vi "rerunSummary.vi"() -> ()   [LabVIEW 2012]
uses:
  <vilib>/addons/database/Auxilliary.llb/DB Tools Cursor Type.ctl
  <vilib>/addons/database/Connection.llb/DB Tools Open Connec (Path).vi
  <vilib>/addons/database/Connection.llb/Conn Execute.vi
  <vilib>/addons/database/Recordset.llb/Rec Destroy - Connection.vi
  <vilib>/addons/database/NI_Database_API.lvlib
panel:
  in  "machine":string
  out "error out":errorcluster
  in  "path":path
  in  "input cluster 2":T1
  out "output cluster":T1
  out "concatenated string":string
  out "concatenated string 2":string
  out "filenames":string[](array[string])
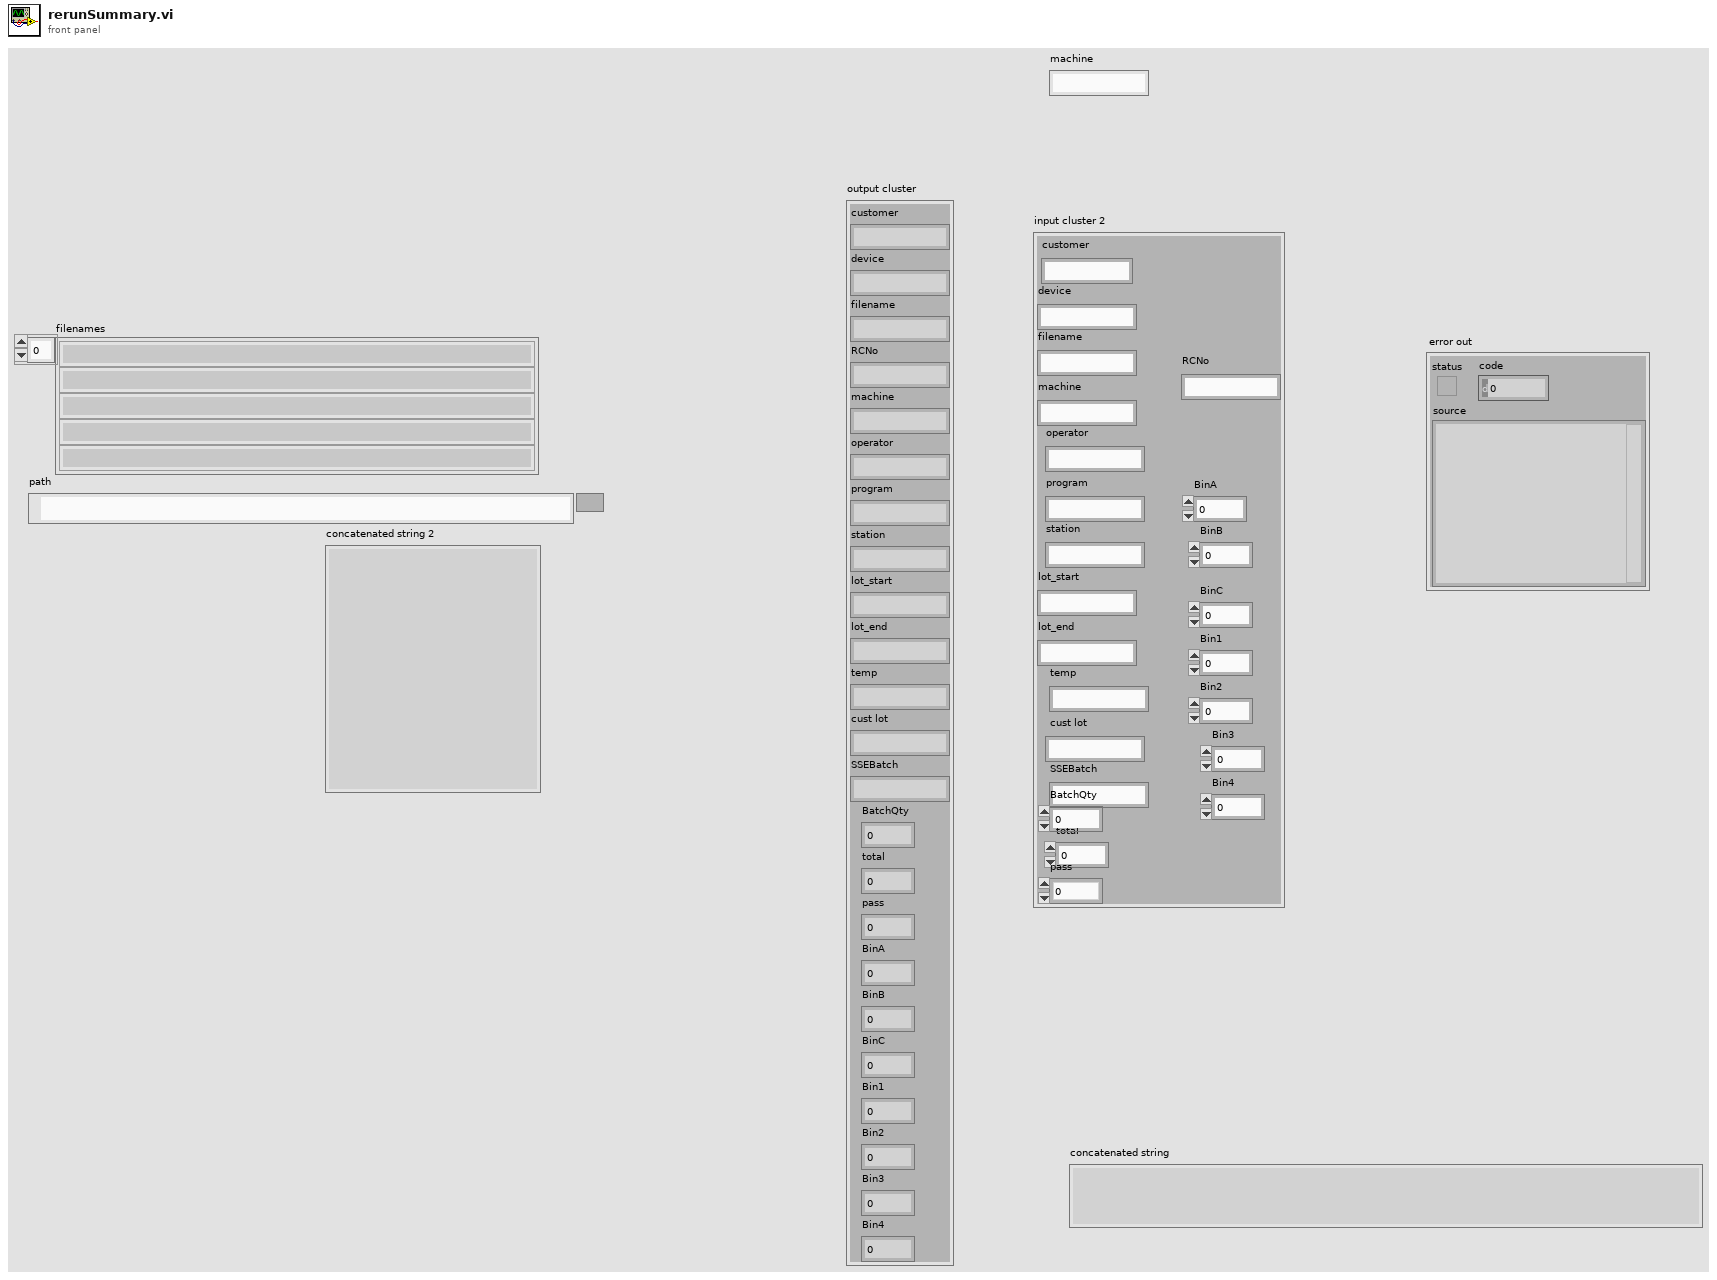
[diagram p1: front panel]
types:
  T1 = cluster{"customer":string, "device":string, "filename":string, "RCNo":string, "machine":string, "operator":string, "program":string, "station":string, "lot_start":string, "lot_end":string, "temp":string, "cust lot":string, "SSEBatch":string, "BatchQty":dbl, "total":dbl, "pass":dbl, "BinA":dbl, "BinB":dbl, "BinC":dbl, "Bin1":dbl, "Bin2":dbl, "Bin3":dbl, "Bin4":dbl}
  T2 = typedef "NI_Database_API.lvlib/Conn ObjectReference.ctl" = refnum<k1>
  T3 = typedef "NI_Database_API.lvlib/DB Tools Cursor Type.ctl" = enum16{"forward-only", "keyset", "dynamic", "static"}
  T4 = typedef "NI_Database_API.lvlib/Rec ObjectReference.ctl" = refnum<k1>
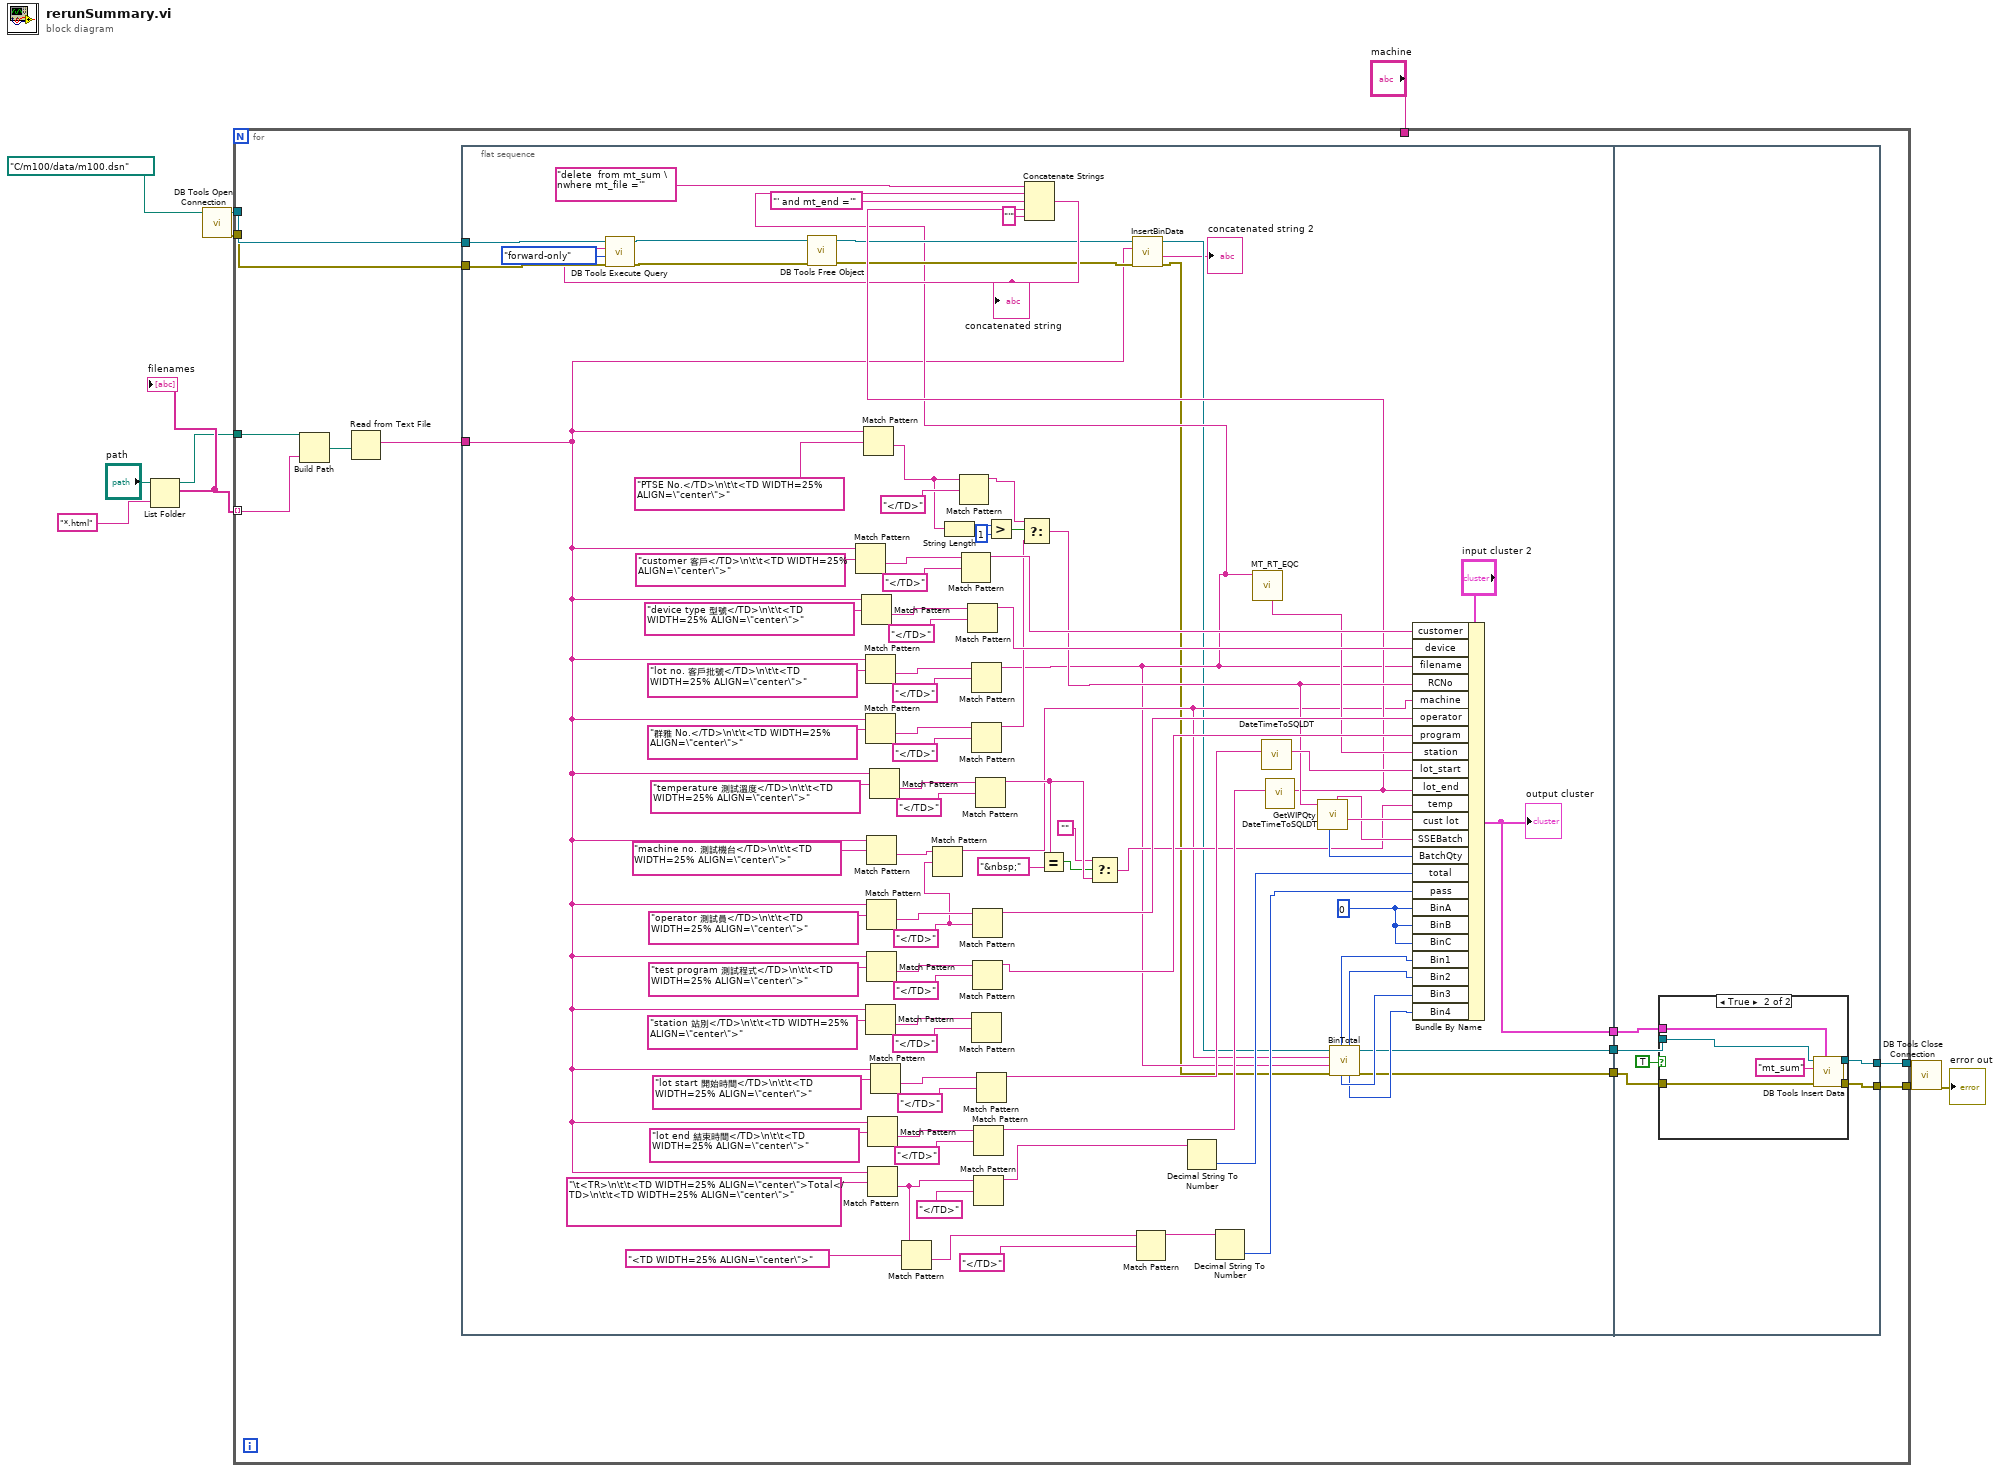
[diagram p0: block diagram]
diagram:
  n1 = List Folder(path="path", pattern="*.html") -> (path out=w9:path, filenames=w10:string[])  [unwired: 2 in, 2 out]
  "filenames" <- w10
  n2 = call-poly <vilib>:"DB Tools Open Connection.vi"("connection information"=path "C:/m100/data/m100.dsn") -> ("error out"=w5:errorcluster, "connection reference"=w6:T2)  [unwired: 7 in]
  n3 = for {
    tunnel: w10 -> [w21] mode=indexing
    tunnel: w9 -> [w20]
    tunnel: w6 -> [w19]
    tunnel: w5 -> [w18]
    tunnel: "machine" -> [_]
    tunnel: [w13] -> w2
    tunnel: [w12] -> w1
    n4 = Build Path(base path=w20, name or relative path=w21) -> (appended path=w22:path)
    n5 = Read from Text File(file (use dialog)=w22) -> (text=w17:string)  [unwired: 3 in, 3 out]
    n6 = flat-sequence {
      tunnel: w19 -> [w56]
      tunnel: w18 -> [w55]
      tunnel: w17 -> [w27]
      tunnel: [w31] -> w16
      tunnel: [w30] -> w15
      tunnel: [w29] -> w14
      tunnel: w16 -> [w122]
      tunnel: w15 -> [w121]
      tunnel: w14 -> [w120]
      tunnel: [w119] -> w13
      tunnel: [w118] -> w12
      frame #0 {
        w28 = 0
        w42 = "</TD>" ("regular expression")
        n7 = Match Pattern(string=w27, regular expression="customer 客戶</TD>\n\t\t<TD WIDTH=25% ALIGN=\"center\">") -> (after substring=w115:string)  [unwired: 1 in, 3 out]
        n8 = Match Pattern(string=w27, regular expression="device type 型號</TD>\n\t\t<TD WIDTH=25% ALIGN=\"center\">") -> (after substring=w112:string)  [unwired: 1 in, 3 out]
        n9 = Match Pattern(string=w27, regular expression="PTSE No.</TD>\n\t\t<TD WIDTH=25% ALIGN=\"center\">") -> (after substring=w72:string)  [unwired: 1 in, 3 out]
        n10 = Match Pattern(string=w27, regular expression="lot no. 客戶批號</TD>\n\t\t<TD WIDTH=25% ALIGN=\"center\">") -> (after substring=w109:string)  [unwired: 1 in, 3 out]
        n11 = Match Pattern(string=w27, regular expression="群雅 No.</TD>\n\t\t<TD WIDTH=25% ALIGN=\"center\">") -> (after substring=w106:string)  [unwired: 1 in, 3 out]
        n12 = Match Pattern(string=w27, regular expression="station 站別</TD>\n\t\t<TD WIDTH=25% ALIGN=\"center\">") -> (after substring=w95:string)  [unwired: 1 in, 3 out]
        n13 = Match Pattern(string=w27, regular expression="machine no. 測試機台</TD>\n\t\t<TD WIDTH=25% ALIGN=\"center\">") -> (after substring=w43:string)  [unwired: 1 in, 3 out]
        n14 = Match Pattern(string=w27, regular expression="operator 測試員</TD>\n\t\t<TD WIDTH=25% ALIGN=\"center\">") -> (after substring=w100:string)  [unwired: 1 in, 3 out]
        n15 = Match Pattern(string=w27, regular expression="test program 測試程式</TD>\n\t\t<TD WIDTH=25% ALIGN=\"center\">") -> (after substring=w98:string)  [unwired: 1 in, 3 out]
        n16 = Match Pattern(string=w27, regular expression="lot end 結束時間</TD>\n\t\t<TD WIDTH=25% ALIGN=\"center\">") -> (after substring=w89:string)  [unwired: 1 in, 3 out]
        n17 = Match Pattern(string=w27, regular expression="\t<TR>\n\t\t<TD WIDTH=25% ALIGN=\"center\">Total</TD>\n\t\t<TD WIDTH=25% ALIGN=\"center\">") -> (after substring=w85:string)  [unwired: 1 in, 3 out]
        n18 = Match Pattern(string=w27, regular expression="temperature 測試溫度</TD>\n\t\t<TD WIDTH=25% ALIGN=\"center\">") -> (after substring=w103:string)  [unwired: 1 in, 3 out]
        n19 = Match Pattern(string=w27, regular expression="lot start 開始時間</TD>\n\t\t<TD WIDTH=25% ALIGN=\"center\">") -> (after substring=w92:string)  [unwired: 1 in, 3 out]
        n20 = Match Pattern(string=w85, regular expression="<TD WIDTH=25% ALIGN=\"center\">") -> (after substring=w82:string)  [unwired: 1 in, 3 out]
        n21 = Match Pattern(string=w43, regular expression=w42) -> (before substring=w35:string)  [unwired: 1 in, 3 out]
        n22 = String Length(string=w72) -> (length=w70:i32)
        n23 = Match Pattern(string=w72, regular expression="</TD>") -> (before substring=w68:string)  [unwired: 1 in, 3 out]
        n24 = Match Pattern(string=w115, regular expression="</TD>") -> (before substring=w79:string)  [unwired: 1 in, 3 out]
        n25 = Match Pattern(string=w112, regular expression="</TD>") -> (before substring=w78:string)  [unwired: 1 in, 3 out]
        n26 = Match Pattern(string=w109, regular expression="</TD>") -> (before substring=w34:string)  [unwired: 1 in, 3 out]
        n27 = Match Pattern(string=w106, regular expression="</TD>") -> (before substring=w67:string)  [unwired: 1 in, 3 out]
        n28 = Match Pattern(string=w95, regular expression="</TD>") -> ()  [unwired: 1 in, 4 out]
        n29 = Match Pattern(string=w100, regular expression=w42) -> (before substring=w77:string)  [unwired: 1 in, 3 out]
        n30 = Match Pattern(string=w98, regular expression="</TD>") -> (before substring=w76:string)  [unwired: 1 in, 3 out]
        n31 = Match Pattern(string=w89, regular expression="</TD>") -> (before substring=w64:string)  [unwired: 1 in, 3 out]
        n32 = Match Pattern(string=w85, regular expression="</TD>") -> (before substring=w81:string)  [unwired: 1 in, 3 out]
        n33 = Match Pattern(string=w103, regular expression="</TD>") -> (before substring=w46:string)  [unwired: 1 in, 3 out]
        n34 = Match Pattern(string=w92, regular expression="</TD>") -> (before substring=w66:string)  [unwired: 1 in, 3 out]
        n35 = Greater?(x=w70, y=1) -> (0:w71:bool)
        n36 = Select(t=w68, s=w71, f=w67) -> (s? t:f=w62:string)
        n37 = Equal?(x=w46, y="&nbsp;") -> (x = y?=w45:bool)
        n38 = Select(t="", s=w45, f=w46) -> (s? t:f=w47:string)
        n39 = Match Pattern(string=w82, regular expression="</TD>") -> (before substring=w75:string)  [unwired: 1 in, 3 out]
        n40 = Decimal String To Number(string=w81) -> (number=w59:i32)  [unwired: 2 in, 1 out]
        n41 = Decimal String To Number(string=w75) -> (number=w60:i32)  [unwired: 2 in, 1 out]
        n42 = call "MT_RT_EQC.vi"("input string"=w34) -> ("STN"=w63:string)  [unwired: 6 in, 4 out]
        n43 = call "DateTimeToSQLDT.vi"("DateTimeString"=w66) -> ("SQLDateTime"=w65:string)  [unwired: 10 in]
        n44 = call "DateTimeToSQLDT.vi"("DateTimeString"=w64) -> ("SQLDateTime"=w52:string)  [unwired: 10 in]
        n45 = Concatenate Strings("delete  from mt_sum \nwhere mt_file ='" ("SQL query"), w34, "' and mt_end ='" ("string"), w52, "'" ("string")) -> (w50:string)
        "concatenated string" <- w50
        n46 = call-poly <vilib>:"DB Tools Execute Query.vi"("error in (no error)"=w55, "cursor type"=DB_Tools_Cursor_Type."forward-only", "SQL query"=w50, "connection reference"=w56) -> ("error out"=w23:errorcluster, "recordset reference"=w24:T4)  [unwired: 4 in]
        n47 = call-poly <vilib>:"DB Tools Free Object.vi"("error in (no error)"=w23, "recordset reference"=w24) -> ("error out"=w40:errorcluster, "connection reference"=w41:T2)  [unwired: 8 in]
        n48 = call "InsertBinData.vi"("error in (no error)"=w40, "string"=w27, "connection reference"=w41) -> ("error out"=w33:errorcluster, "concatenated string"=→"concatenated string 2":string, "connection reference out"=w32:T2)  [unwired: 6 in]
        n49 = call "GetWIPQty.vi"("Lotno"=w62) -> ("lotno"=w61:string, "SSEBATCH"=w57:string, "BATCHQTY"=w58:i32)  [unwired: 3 in, 5 out]
        n50 = call "BinTotal.vi"("error out 2"=w33, "fileName"=w34, "machine"=w35, "connection reference"=w32) -> ("error out"=w30:errorcluster, "connection reference 2"=w31:T2, "bin4"=w36:i32, "bin2"=w38:i32, "bin3"=w37:i32, "bin1"=w39:i32)  [unwired: 2 in]
        n51 = Bundle By Name(cluster="input cluster 2", "customer"=w79, "device"=w78, "filename"=w34, "RCNo"=w62, "machine"=w35, "operator"=w77, "program"=w76, "station"=w63, "lot_start"=w65, "lot_end"=w52, "temp"=w47, "cust lot"=w61, "SSEBatch"=w57, "BatchQty"=w58, "total"=w59, "pass"=w60, "BinA"=w28, "BinB"=w28, "BinC"=w28, "Bin1"=w39, "Bin2"=w38, "Bin3"=w37, "Bin4"=w36) -> (w29:T1)
        "output cluster" <- w29
      }
      frame #1 {
        n52 = case shown="True" TRUE {
          tunnel: [w124 w130] -> w119
          tunnel: [w123 w129] -> w118
          tunnel: w122 -> [w124 w127]
          tunnel: w121 -> [w123 w126]
          tunnel: w120 -> [_ w125]
          frame False {
          }
          frame True {
            n53 = call <vilib>:"DB Tools Insert Data.vi"("data"=w125, "error in (no error)"=w126, "table"="mt_sum", "connection reference"=w127) -> ("error out"=w129:errorcluster, "connection reference out"=w130:T2)  [unwired: 6 in]
          }
        }
      }
    }
  }
  n54 = call <vilib>:"DB Tools Close Connection.vi"("error in (no error)"=w1, "connection reference"=w2) -> ("error out"=→"error out":errorcluster)  [unwired: 5 in]
